vi "CSM-Name to CSM-Mode.vi"(11 "String":string) -> (1 "ParentCSM Name":string, 2 "CSM Mode":T1, 3 "Requested Name":string)   [LabVIEW 2020, in "Communicable State Machine.lvlib"]
uses:
  Communicable State Machine.lvlib
  _CSM_NAME_REQUEST.ctl
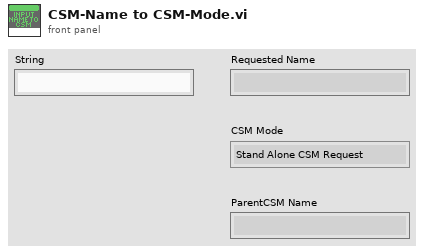
[diagram p1: front panel]
types:
  T1 = typedef "Communicable State Machine.lvlib/_CSM_NAME_REQUEST.ctl" = enum16{"Stand Alone CSM Request", "Normal CSM Request", "Agent Request", "Action Worker Request", "Chain Request", "Chain Node Request"}
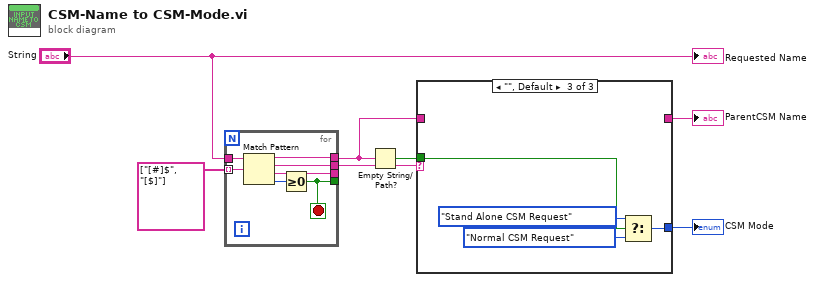
[diagram p0: block diagram]
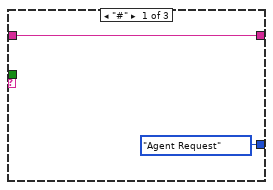
[diagram p2: hidden frame]
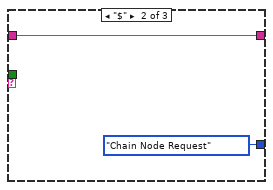
[diagram p3: hidden frame]
diagram:
  n1 = for {
    tunnel: "String" -> [w14]
    tunnel: string[] ["[#]$", "[$]"] -> [w13] mode=indexing
    tunnel: [w11] -> _
    tunnel: [w10] -> w3
    tunnel: [w9] -> w6
    tunnel: [w8] -> _
    stop <- w11 stop-if-true
    n2 = Match Pattern(string=w14, regular expression=w13) -> (before substring=w10:string, match substring=w9:string, after substring=w8:string, offset past match=w12:i32)  [unwired: 1 in]
    n3 = Greater Or Equal To 0?(x=w12) -> (x >= 0?=w11:bool)
  }
  n4 = Empty String/Path?(string/path=w3) -> (empty?=w4:bool)
  n5 = case shown="\"\", Default" w6 {
    tunnel: [_CSM_NAME_REQUEST."Agent Request" ("CSM Mode") _CSM_NAME_REQUEST."Chain Node Request" ("CSM Mode") w21] -> w5
    tunnel: w4 -> [_ _ w19]
    tunnel: w3 -> [w15 w17 _]
    tunnel: [w15 w17 _] -> w1
    frame "#" {
    }
    frame "$" {
    }
    frame "", Default {
      n6 = Select(t=_CSM_NAME_REQUEST."Stand Alone CSM Request" ("CSM Mode"), s=w19, f=_CSM_NAME_REQUEST."Normal CSM Request" ("CSM Mode")) -> (s? t:f=w21:T1)
    }
  }
  "CSM Mode" <- w5
  "ParentCSM Name" <- w1
  "Requested Name" <- "String"
